vi "Wyznaczanie spektrum amplitudowego.vi"(11 "signal in":waveform(dbl)) -> (1 "As2":dbl[](array[numeric]), 2 "As":dbl[](array[numeric]), 3 "Waveform Graph":waveform(dbl)(graph), 4 "Waveform":waveform(dbl), 5 "N2":dbl, 6 "df":dbl)   [LabVIEW 2025]
uses:
  <vilib>/Analysis/2dsp.llb/Real FFT.vi
  <vilib>/Analysis/NI_AALPro.lvlib
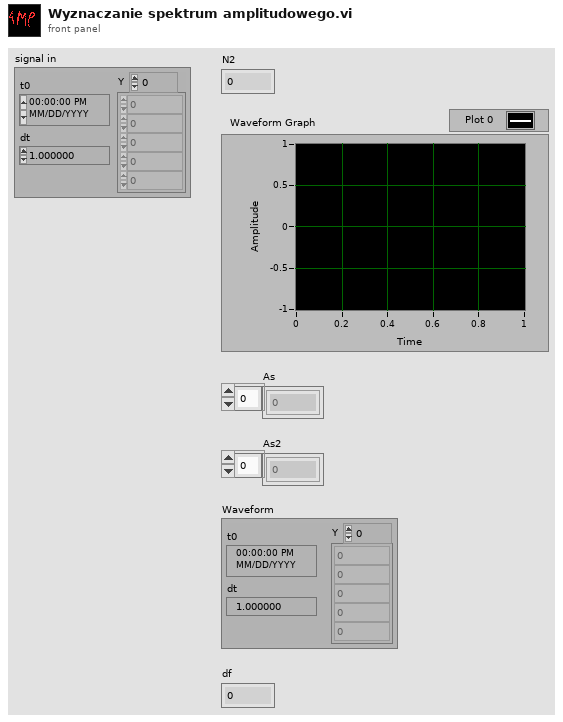
[diagram p1: front panel]
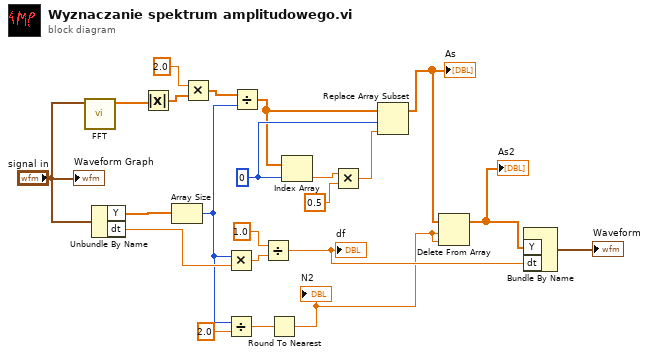
[diagram p0: block diagram]
diagram:
  w10 = 0 ("index")
  n1 = call-poly <vilib>:"FFT.vi"("X"="signal in") -> ("FFT {X}"=w4:cdb[])  [unwired: 9 in, 1 out]
  n2 = Unbundle By Name("signal in") -> ("Y"=w1:dbl[], "dt"=w22:dbl)
  n3 = Absolute Value(x=w4) -> (abs(x)=w5:dbl[])
  n4 = Array Size(array=w1) -> (size(s)=w16:i32)
  n5 = Multiply(x=2.0, y=w5) -> (x*y=w6:dbl[])
  n6 = Multiply(x=w16, y=w22) -> (x*y=w13:dbl)
  n7 = Divide(x=w16, y=2.0) -> (x/y=w14:dbl)
  n8 = Divide(x=w6, y=w16) -> (x/y=w9:dbl[])
  n9 = Divide(x=1.0, y=w13) -> (x/y=w20:dbl)
  "df" <- w20
  n10 = Round To Nearest(number=w14) -> (nearest integer value=w18:dbl)
  "N2" <- w18
  n11 = Index Array(array=w9, index=w10) -> (element=w7:dbl)
  n12 = Multiply(x=w7, y=0.5) -> (x*y=w11:dbl)
  n13 = Replace Array Subset(array=w9, new element=w11, index=w10) -> (w17:dbl[])
  "As" <- w17
  n14 = Delete From Array(array=w17, length=w18, index=w18) -> (array with subset deleted=w19:dbl[])  [unwired: 1 out]
  "As2" <- w19
  n15 = Bundle By Name("Y"=w19, "dt"=w20) -> (→"Waveform":waveform(dbl))  [unwired: 1 in]
  "Waveform Graph" <- "signal in"
